vi "GPIB Error Report.vi"(2 "Boolean":bool, 4 "Function":string="A GPIB function ", 5 "Dialog?(F)":bool, 6 "Status":bool[](array[boolean])=[FALSE, FALSE, FALSE, FALSE, FALSE, FALSE, FALSE, FALSE, FALSE, FALSE, FALSE, FALSE, FALSE, FALSE, FALSE, FALSE], 7 "Address String":string) -> (0 "Error String":string, 1 "Status String":string)   [LabVIEW 2022 SP3]
doc: "Interpret the Status bits returned by a GPIB function and report the status and any error as text. If Dialog is True, the error message will be reported in a dialog box, and the user will have the choice of aborting or continuing."
panel:
  in  "Error strings":string[](array[string])=["EDVR:  Error connecting to driver or device.", "ECIC - Command requires GPIB controller to be CIC", "ENOL - Write detected no listeners", "EADR - GPIB controller not addressed correctly", "EARG - Invalid argument or arguments", "ESAC - Command requires GPIB controller to be system controller", "EABO - I/O operation aborted", "ENEB - Non-existent board", "EDMA - DMA hardware error detected", "EBTO - DMA hardware uP bus timeout", "EOIP - New I/O attempted with old I/O in progress", "ECAP - No capability for operation", "EFSO - File system operation error", "EOWN - Sharable board exclusively owned", "TIMO - Timeout", "ESTB - Serial poll byte queue overflow", "ESRQ - SRQ stuck on", "ECMD - Unrecognized command", "", "EBNP - Board not present", "EINTRP - Interpreter error (MacBus)", "", "", "", "", "", "", "", "", "", "NADDR - No GPIB address input", "NSTRG - No string input (write)", "NCNT - No count input (read)", "", "", "", "", "", "", "", "EMOM - Out of memory (MacBus)", "EMIM - Insufficient memory (MacBus)", "", "", "", "", "", "", "", "", "ECOMM - Breakdown in SCSI protocols (MacBus)", "", "", "", "", "", "", "", "", "", "", "EPAR - Serial port parity error", "EORN - Serial port overrun error", "EOFL - Serial port receive buffer overflow", "EFRM - Serial port framing error", "SPTMO - Serial port timeout, bytes not received at serial port"]
  in  "Status bit strings":string[](array[string])=["DCAS - Device Clear State", "DTAS - Device Trigger State", "LACS - Listener Active State", "TACS - Talker Active State", "ATN - Attention Asserted", "CIC - Controller In Charge", "REM - Remote State", "LOK - Lockout State", "CMPL - Operation Completed", "", "", "", "SRQI - SRQ detected while CIC", "END - EOI or EOS detected", "TIMO - Timeout", "ERR - Error Detected"]
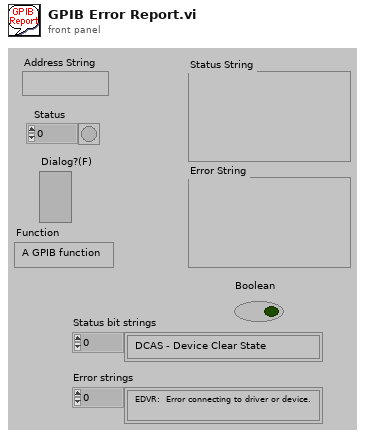
[diagram p1: front panel]
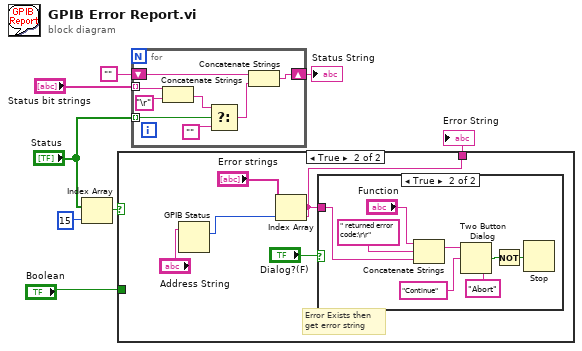
[diagram p0: block diagram]
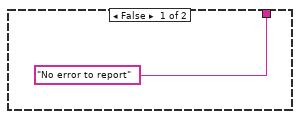
[diagram p2: hidden frame]
diagram:
  n1 = Index Array(array="Status", index=15) -> (element=w3:bool)
  n2 = case shown="True" w3 {
    tunnel: ["No error to report" w11] -> w2
    tunnel: "Boolean" -> [_ _]
    frame False {
    }
    frame True {
      # "Error Exists then get error string"
      n3 = GPIB Status(0:"Address String") -> (3:w13:i16)  [unwired: 1 in, 3 out]
      n4 = Index Array(array="Error strings", index=w13) -> (element=w11:string)
      n5 = case shown="True" "Dialog?(F)" {
        tunnel: w11 -> [_ w15]
        frame False {
        }
        frame True {
          n6 = Concatenate Strings("Function", " returned error code:\r\r", w15) -> (w21:string)
          n7 = Two Button Dialog(message=w21, 1:"Abort", 2:"Continue") -> (T button?=w18:bool)
          n8 = Not(x=w18) -> (.not. x?=w17:bool)
          n9 = Stop(stop? (T)=w17) -> ()
        }
      }
    }
  }
  "Error String" <- w2
  n10 = for {
    shift-right: [w23] -> w6
    shift-left: "" -> [w25]
    tunnel: "Status" -> [w28] mode=indexing
    tunnel: "Status bit strings" -> [w30] mode=indexing
    n11 = Concatenate Strings(w30, "\r") -> (w27:string)
    n12 = Select(t=w27, s=w28, f="") -> (s? t:f=w24:string)
    n13 = Concatenate Strings(w25, w24) -> (w23:string)
  }
  "Status String" <- w6
